vi "ThresholdImage.vi"(0 "Method":i32(ring) items=["Niblack", "Background Correction", "Constant Threshold", "Auto Threshold"], 1 "Image Src":T1, 2 "Cluster":T4={"Look for"=0, "Window Size(32x32)"={"SizeX"=32, "SizeY"=32}, "Niblack Deviation Factor"=0.2, "Range"={"Lower value"=128, "Upper value"=255}, "Number of Erosion"=2} {"Range"."Upper value" scale=0.0..255.0; "Range"."Lower value" scale=0.0..255.0; "Niblack Deviation Factor" min=0.0 max=1.0 format="%.2f"; "Window Size(32x32)"."SizeY" min=3 step=1; "Window Size(32x32)"."SizeX" min=3 step=1; "Look for" items=["Bright Objects", "Dark Objects"]}, 3 "ROI Descriptor":T2 {"Contours"."Type" items=["No Selection", "Point", "Line", "Rectangle", "Oval", "Polygon", "Freehand Region", "Annulus", "Unused2", "Unused3", "Broken Line", "Freehand Line", "Rotated Rectangle"]}) -> (7 "Clamp Results":T3, 8 "Threshold":T1, 9 "Improved Threshold":T1, 10 "Clamped Image":T1)   [LabVIEW 2015]
uses:
  <vilib>/vision/Image Controls.llb/IMAQ Image.ctl
  <vilib>/vision/NI_Vision_Development_Module.lvlib
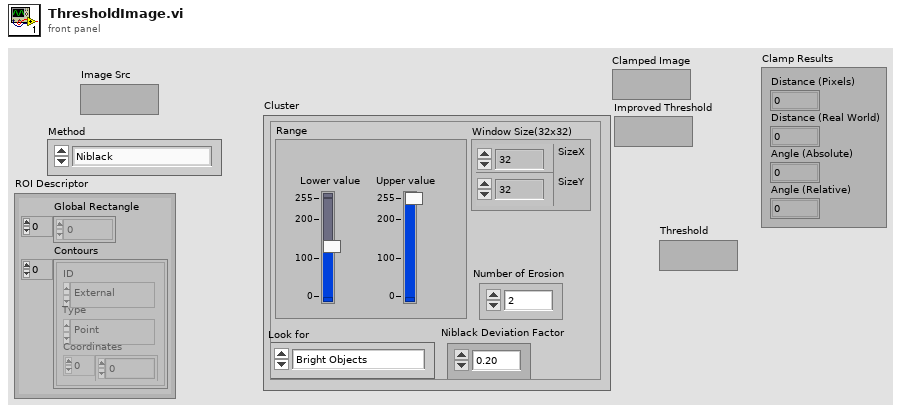
[diagram p1: front panel]
types:
  T1 = typedef "IMAQ Image.ctl" = refnum<image>
  T2 = typedef "ROI Descriptor" = cluster{"Global Rectangle":i32[], "Contours":cluster{"ID":enum32{"External", "Internal"}, "Type":u32, "Coordinates":i32[]}[]}
  T3 = cluster{"Distance (Pixels)":dbl, "Distance (Real World)":dbl, "Angle (Absolute)":dbl, "Angle (Relative)":dbl}
  T4 = cluster{"Look for":i32, "Window Size(32x32)":cluster{"SizeX":i32, "SizeY":i32}, "Niblack Deviation Factor":dbl, "Range":cluster{"Lower value":i32, "Upper value":i32}, "Number of Erosion":i32}
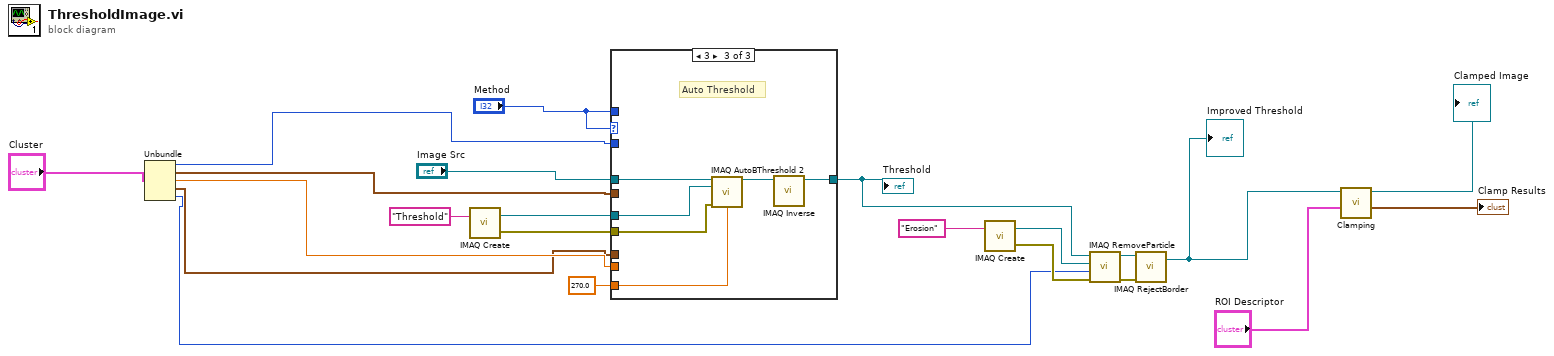
[diagram p0: block diagram]
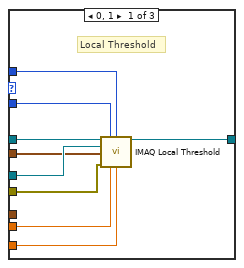
[diagram p2: hidden frame]
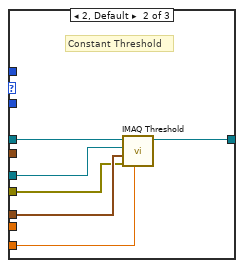
[diagram p3: hidden frame]
diagram:
  n1 = Unbundle("Cluster") -> ("Look for"=w9:i32, "Window Size(32x32)"=w8:cluster{"SizeX":i32, "SizeY":i32}, "Niblack Deviation Factor"=w7:dbl, "Range"=w6:cluster{"Lower value":i32, "Upper value":i32}, "Number of Erosion"=w5:i32)
  n2 = call "IMAQ Create"("Image Name"="Threshold") -> ("New Image"=w21:T1, "error out"=w19:errorcluster)  [unwired: 4 in]
  n3 = case shown="3" "Method" {
    tunnel: "Method" -> [w31 _ _]
    tunnel: w9 -> [w30 _ _]
    tunnel: w21 -> [w28 w37 w41]
    tunnel: w6 -> [_ w36 _]
    tunnel: "Image Src" -> [w29 w35 w43]
    tunnel: [w27 w34 w38] -> w12
    tunnel: sgl 270.0 ("Replace Value") -> [w26 w33 w42]
    tunnel: w7 -> [w25 _ _]
    tunnel: w19 -> [w24 w32 w40]
    tunnel: w8 -> [w23 _ _]
    frame 0, 1 {
      # "Local Threshold"
      n4 = call "IMAQ Local Threshold"("Image Src"=w29, "Look For (Bright Objects)"=w30, "Method (Niblack)"=w31, "Image Dst"=w28, "Window Size (32x32)"=w23, "error in (no error)"=w24, "Niblack Deviation Factor (0.2)"=w25, "Replace Value (1)"=w26) -> ("Image Dst Out"=w27:T1)  [unwired: 6 in, 1 out]
    }
    frame 2, Default {
      # "Constant Threshold"
      n5 = call "IMAQ Threshold"("Replace Value"=w33, "error in (no error)"=w32, "Range"=w36, "Image Dst"=w37, "Image Src"=w35) -> ("Image Dst Out"=w34:T1)  [unwired: 5 in, 1 out]
    }
    frame 3 {
      # "Auto Threshold"
      n6 = call "IMAQ AutoBThreshold 2"("Image Src"=w43, "Image Dst"=w41, "error in (no error)"=w40, "Replace Value (1)"=w42) -> ("Image Dst Out"=w39:T1)  [unwired: 9 in, 2 out]
      n7 = call "IMAQ Inverse"("Image Src"=w39) -> ("Image Dst Out"=w38:T1)  [unwired: 9 in, 1 out]
    }
  }
  "Threshold" <- w12
  n8 = call "IMAQ Create"("Image Name"="Erosion") -> ("New Image"=w15:T1, "error out"=w13:errorcluster)  [unwired: 4 in]
  n9 = call "IMAQ RemoveParticle"("error in (no error)"=w13, "Number of Erosion"=w5, "Image Dst"=w15, "Image Src"=w12) -> ("error out"=w14:errorcluster, "Image Dst Out"=w17:T1)  [unwired: 6 in]
  n10 = call "IMAQ RejectBorder"("error in (no error)"=w14, "Image Src"=w17) -> ("Image Dst Out"=w1:T1)  [unwired: 4 in, 1 out]
  "Improved Threshold" <- w1
  n11 = call "Clamping.vi"("Source Image"=w1, "ROI Descriptor"="ROI Descriptor") -> ("Image Out"=→"Clamped Image":T1, "Clamp Results"=→"Clamp Results":T3)  [unwired: 7 in]
